vi "FindBlob_Count.vi"(1 "Image Data in":u32[](array[numeric])) -> (2 "Image Data out":u32[](graph), 3 "Area (pixels)":i32[](array[numeric]), 4 "# particles":i32)   [LabVIEW 2024]
uses:
  <vilib>/Analysis/NI_AALPro.lvlib
panel:
  out "Histogram":T1(graph)
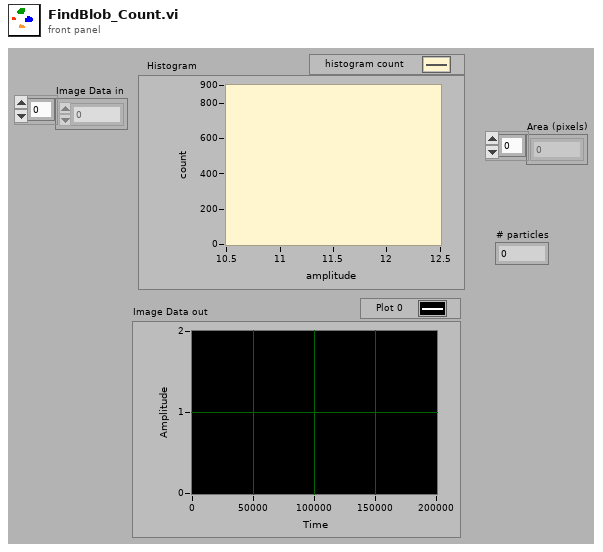
[diagram p1: front panel]
types:
  T1 = cluster{"X Values":dbl[], "Histogram: h(x)":i32[]}
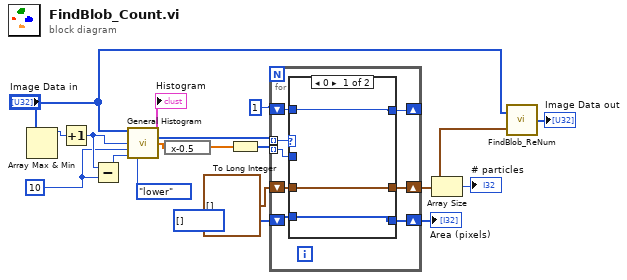
[diagram p0: block diagram]
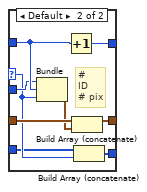
[diagram p2: hidden frame]
diagram:
  w1 = u8 10 ("min")
  n1 = Array Max & Min(array="Image Data in") -> (max value=w8:u32)  [unwired: 3 out]
  n2 = Increment(x=w8) -> (x+1=w2:u32)
  n3 = Subtract(x=w2, y=w1) -> (x-y=w7:u32)
  n4 = call <vilib>:"General Histogram.vi"("X"="Image Data in", "max"=w2, "min"=w1, "# bins"=w7, "inclusion"=enum32{"lower", "upper"}."lower") -> ("Histogram Graph"=→"Histogram":T1, "Histogram"=w15:i32[], "Axis"=w6:dbl[])  [unwired: 1 in, 7 out]
  n5 = expression code="x-0.5"(w6) -> (w5:dbl[])
  n6 = To Long Integer(number=w5) -> (32bit integer=w9:i32[])
  n7 = for {
    tunnel: w15 -> [w26] mode=indexing
    tunnel: w9 -> [w23] mode=indexing
    shift-right: [w21] -> w12
    shift-left: cluster{u8, i32, i32}[] [] -> [w22]
    shift-right: [w24] -> _
    shift-left: u8 1 -> [w25]
    shift-right: [w19] -> w3
    shift-left: i32[] [] -> [w20]
    n8 = case shown="0" w26 {
      selector: w26 -> [_ w32]
      tunnel: w25 -> [w29 w34]
      tunnel: [w29 w38] -> w24
      tunnel: w23 -> [_ w33]
      tunnel: w22 -> [w28 w37]
      tunnel: [w28 w35] -> w21
      tunnel: w20 -> [w27 w31]
      tunnel: [w27 w30] -> w19
      frame 0 {
      }
      frame Default {
        # "#\nID\n# pix"
        n9 = Bundle(w33, w34, w32) -> (w36:cluster{i32, u8, i32})  [unwired: 1 out]
        n10 = Increment(x=w34) -> (x+1=w38:u8)
        n11 = Build Array (concatenate)(w37, w36) -> (w35:cluster{i32, i32, i32}[])
        n12 = Build Array (concatenate)(w31, w32) -> (w30:i32[])
      }
    }
  }
  "Area (pixels)" <- w3
  n13 = Array Size(array=w12) -> (size(s)=→"# particles":i32)
  n14 = call <userlib>:"FindBlob_ReNum.vi"("duplicates"=w12, "Image Data in"="Image Data in") -> ("Image Data out"=→"Image Data out":u32[])
